vi "Double-Click Action.vi"(7 "Device Ref in":T2 format="%.0x", 8 "error in (no error)":errorcluster, 9 "Mods.Double Click":bool, 10 "Coords":T1, 11 "CtlRef":refnum<vi>) -> (0 "error out":errorcluster)   [LabVIEW 2014, in "SLSC configuration System Explorer.lvlib"]
uses:
  SLSC configuration System Explorer.lvlib
  <vilib>/NI Veristand/Custom Device API/Custom Device Item Ref.ctl
  <vilib>/Utility/miscctls.llb/LVPoint32TypeDef.ctl
  <vilib>/NI Veristand/Custom Device Tools/Custom Device Utility Library/NI VeriStand - Search for Item by Name.vi
  <vilib>/NI Veristand/Custom Device Tools/Custom Device Utility Library/Custom Device Utility Library.lvlib
  <vilib>/NI Veristand/Custom Device API/Custom Device API.lvlib
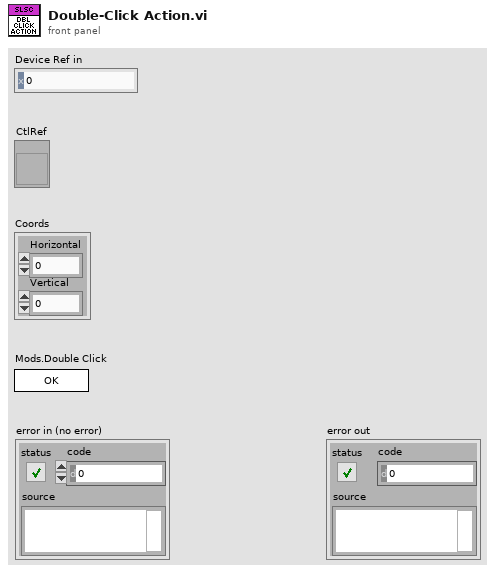
[diagram p1: front panel]
types:
  T1 = typedef "LVPoint32TypeDef.ctl" = cluster{"Horizontal":i32, "Vertical":i32}
  T2 = typedef "Custom Device API.lvlib/Custom Device Item Ref.ctl" = u64
  T3 = typedef "LVRowAndColumnTypeDef.ctl" = cluster{"Row":i32, "Column":i32}
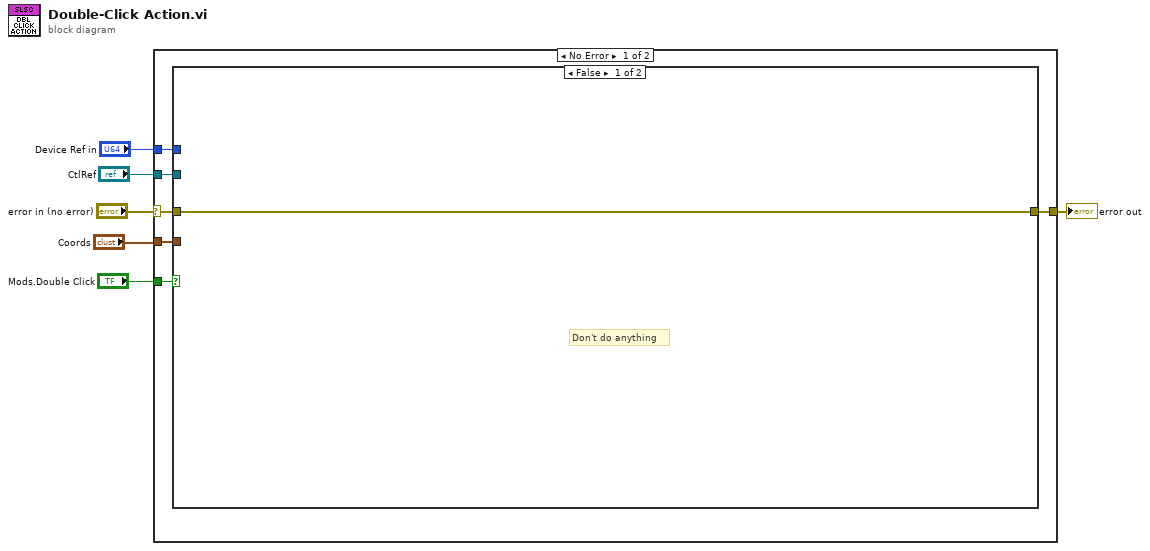
[diagram p0: block diagram]
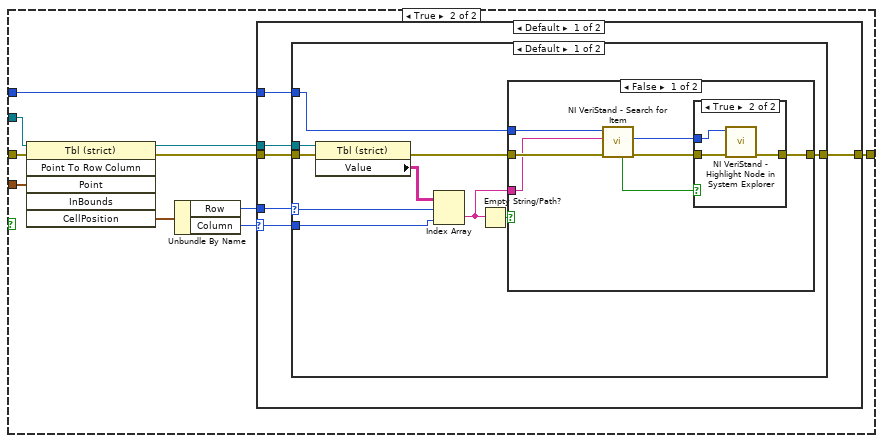
[diagram p2: hidden frame]
diagram:
  n1 = case shown="No Error" "error in (no error)" {
    selector: "error in (no error)" -> [w10 w54]
    tunnel: "Coords" -> [w12 _]
    tunnel: "CtlRef" -> [w11 _]
    tunnel: "Device Ref in" -> [w9 _]
    tunnel: [w8 w54] -> w3
    tunnel: "Mods.Double Click" -> [w7 _]
    frame No Error {
      n2 = case shown="False" w7 {
        tunnel: w12 -> [_ w23]
        tunnel: w11 -> [_ w22]
        tunnel: w10 -> [w13 w21]
        tunnel: w9 -> [_ w15]
        tunnel: [w13 w14] -> w8
        frame False {
          # "Don't do anything"
        }
        frame True {
          n3 = invoke class="Tbl (strict)" method="Point To Row Column"(reference=w22, error in=w21, "Point"=w23) -> (reference out=w16:refnum<vi>, error out=w17:errorcluster, "CellPosition"=w20:T3)  [unwired: 3 in, 3 out]
          n4 = Unbundle By Name(w20) -> ("Row"=w18:i32, "Column"=w19:i32)
          n5 = case shown="Default" w19 {
            selector: w19 -> [w26 _]
            tunnel: w18 -> [w29 _]
            tunnel: w17 -> [w28 w53]
            tunnel: w16 -> [w27 _]
            tunnel: w15 -> [w25 _]
            tunnel: [w24 w53] -> w14
            frame Default {
              n6 = case shown="Default" w29 {
                selector: w29 -> [w36 _]
                tunnel: w28 -> [w39 w52]
                tunnel: w27 -> [w38 _]
                tunnel: w26 -> [w35 _]
                tunnel: w25 -> [w31 _]
                tunnel: [w30 w52] -> w24
                frame Default {
                  n7 = property class="Tbl (strict)"(reference=w38, error in=w39) -> (error out=w32:errorcluster, "Value"=w37:string[][])  [unwired: 1 out]
                  n8 = Index Array(array=w37, index (row)=w36, index (col)=w35) -> (element=w33:string)
                  n9 = Empty String/Path?(string/path=w33) -> (empty?=w34:bool)
                  n10 = case shown="False" w34 {
                    tunnel: w33 -> [w44 _]
                    tunnel: w32 -> [w46 w51]
                    tunnel: w31 -> [w45 _]
                    tunnel: [w41 w51] -> w30
                    frame False {
                      n11 = call-poly <vilib>:"NI VeriStand - Search for Item.vi"("error in"=w46, "Item Name"=w44, "Section Ref in"=w45) -> ("error out"=w43:errorcluster, "Item Ref"=w42:T2, "Found"=w40:bool)  [unwired: 5 in, 1 out]
                      n12 = case shown="True" w40 {
                        tunnel: w43 -> [w47 w50]
                        tunnel: w42 -> [_ w49]
                        tunnel: [w47 w48] -> w41
                        frame False {
                        }
                        frame True {
                          n13 = call <vilib>:"NI VeriStand - Highlight Node in System Explorer.vi"("error in (no error)"=w50, "Item Ref in"=w49) -> ("error out"=w48:errorcluster)  [unwired: 8 in, 1 out]
                        }
                      }
                    }
                    frame True {
                      # "Don't do anything"
                    }
                  }
                }
                frame 0 {
                  # "Don't do anything"
                }
              }
            }
            frame 0, 1 {
              # "Don't do anything"
            }
          }
        }
      }
    }
    frame Error {
    }
  }
  "error out" <- w3
